vi "SVX Waterfall Create Lines.vi"   [LabVIEW 2017]
doc: "Creates a line that can be plotted on a waterfall graph. Use the waterfall graph property node \"lines\" to draw the line on the graph."
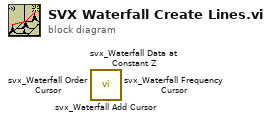
[diagram p0: block diagram]
diagram:
  n1 = call <vilib>:"svx_Waterfall Add Cursor.vi"() -> ()  [unwired: 16 in, 4 out]
  n2 = call <vilib>:"svx_Waterfall Data at Constant Z.vi"() -> ()  [unwired: 15 in, 5 out]
  n3 = call <vilib>:"svx_Waterfall Order Cursor.vi"() -> ()  [unwired: 14 in, 6 out]
  n4 = call <vilib>:"svx_Waterfall Frequency Cursor.vi"() -> ()  [unwired: 14 in, 6 out]
